vi "ActDriveStraightWeird.vi"(9 "FirstTime":bool, 10 "MaxSpeed (ft/s)":dbl, 11 "Dist (ft)":dbl) -> (1 "XSpeedDemand":dbl, 3 "Done":bool)   [LabVIEW 2020]
doc: "Robot will drive forward straight a set distance utilizing position control \n\nInputs:\n-- MaxSpeed -- Double -- in ft/s, the MaxSpeed the robot can go -- \n-- Dist (ft) -- Double -- Distance in feet you want the robot to go -- \n-- FirstTime -- Boolean -- Input true the first time this function is called, sets the target position -- \n\nOutputs:\n-- Done -- Bool -- has the robot reached its target distance\n-- LeftSpeedDemand -- Double -- Speed Demand for left drive train inorder to reach target -- \n-- RightSpeedDemand -- Double -- Speed Demand for left drive train inorder to reach target --"
uses:
  <vilib>/Rock Robotics/WPI/ThirdParty/JAS_Junk/TrajLib/Trajectory_Library.lvlib
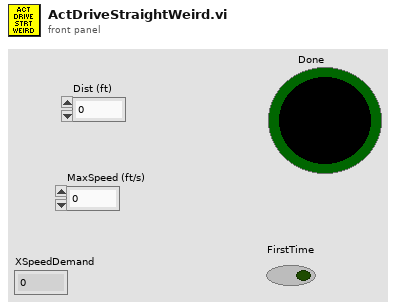
[diagram p1: front panel]
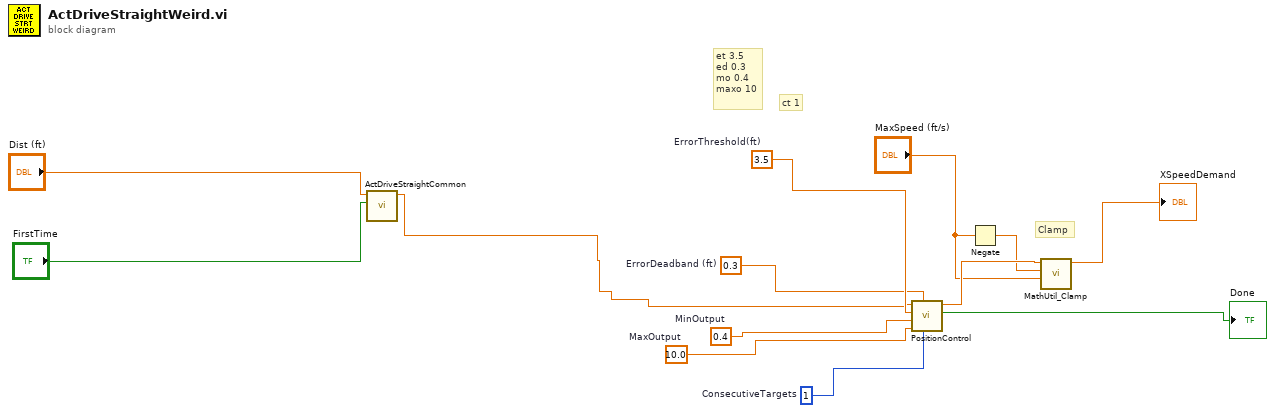
[diagram p0: block diagram]
diagram:
  w8 = 10.0  # MaxOutput
  w7 = 0.4  # MinOutput
  w9 = 1  # ConsecutiveTargets
  w5 = 0.3  # ErrorDeadband (ft)
  w6 = 3.5  # ErrorThreshold(ft)
  # "Clamp"
  # "ct 1"
  # "et 3.5\ned 0.3\nmo 0.4\nmaxo 10"
  n1 = call "ActDriveStraightCommon.vi"("FirstTime"="FirstTime", "Dist (ft)"="Dist (ft)") -> ("Error"=w1:dbl)  [unwired: 9 in]
  n2 = call "PositionControl.vi"("ConsecutiveTargets"=w9, "ErrorDeadband"=w5, "MaxOutput"=w8, "MinOutput"=w7, "ErrorThreshold"=w6, "Error"=w1) -> ("OnTarget"=→"Done":bool, "OutputValue"=w13:dbl)  [unwired: 3 in, 1 out]
  n3 = Negate(x="MaxSpeed (ft/s)") -> (-x=w12:dbl)
  n4 = call <vilib>:"MathUtil_Clamp.vi"("High Limit"="MaxSpeed (ft/s)", "Low Limit"=w12, "Value"=w13) -> ("Result"=→"XSpeedDemand":dbl)  [unwired: 8 in]
